vi "TCP Client_33.vi"(0 "CMD":i32(ring) items=["OCP_IF_CMD_TRACE_READ", "OCP_IF_CMD_TRACE_RESET", "OCP_IF_CMD_TRACE_GET_SIZE", "OCP_IF_CMD_TRACE_SET_SIZE", "OCP_IF_CMD_TRACE_GET_NUMBER_SIGNALS", "OCP_IF_CMD_TRACE_GET_SIGNALS_NAMES", "OCP_IF_CMD_TRACE_GET_NUMBER_TRACES", "OCP_IF_CMD_TRACE_GET_TRACES_NAMES", "OCP_IF_CMD_TRACE_GET_ADDRESS", "OCP_IF_CMD_CS_STATUS", "OCP_IF_CMD_CS_ENABLE", "OCP_IF_CMD_CS_DISABLE", "OCP_IF_CMD_CS_CONTROLLER_IF", "OCP_IF_CMD_CS_HARDWARE_IF", "OCP_IF_CMD_CS_GET_NUMBER_CONTROLLERS", "OCP_IF_CMD_CS_GET_CONTROLLERS_NAMES", "OCP_IF_CMD_PLATFORM_ID", "OCP_IF_CMD_PLATFORM_IF", "OCP_IF_CMD_OPIL_UPDATE_MEASUREMENTS", "OCP_IF_CMD_OPIL_UPDATE_SIM_DATA", "OCP_IF_CMD_OPIL_RUN_CONTROL", "OCP_IF_CMD_OPIL_INITIALIZE_CONTROL", "OCP_IF_CMD_OPIL_GET_CONTROL", "OCP_IF_CMD_OPIL_GET_CONTROLLER_DATA", "OCP_IF_CMD_END"], 2 "Input Cluster":T3, 3 "error in (no error)":errorcluster, 8 "Comunication Cluster":T1) -> (6 "Output cluster":T2, 7 "R_message 1":string, 10 "error out":errorcluster)   [LabVIEW 2021]
uses:
  <vilib>/ErrorRing/Error Ring.xnode
  <vilib>/Utility/error.llb/Error Cluster From Error Code.vi
panel:
  out "R_Data string length":cluster{i32}
  out "W_Data string length: \nbytes written 2":i32
  out "W_Data string_flat":string
  # "0-> OCP_IF_CMD_TRACE_READ = 0, //LV: SIZE - CMD - ID || RESPONSE: SIZE - DATA\n1->\tOCP_IF_CMD_TRACE_RESET, //SIZE - CMD - ID || RESPONSE: SIZE\n2-> OCP_IF_CMD_TRACE_GET_SIZE, //SIZE - CMD - ID || RESPONSE: SIZE - TRACE_SIZE (4 bztes)\n3->\tOCP_IF_CMD_TRACE_SET_SIZE, //SIZE - CMD - ID - TRACE_SIZE ( 4 bytes) || RESPONSE: SIZE\n4->\tOCP_IF_CMD_TRACE_GET_NUMBER_SIGNALS, //SIZE - CMD - ID || RESPONSE: SIZE - NB_SIGNALS (4 bytes)\n5->\tOCP_IF_CMD_TRACE_GET_SIGNALS_NAMES, //SIZE - CMD - ID || RESPONSE: SIZE - string\n6->\tOCP_IF_CMD_TRACE_GET_NUMBER_TRACES, //SIZE - CMD  || RESPONSE: SIZE - NB_TRACES (4 bytes)\n7->\tOCP_IF_CMD_TRACE_GET_TRACES_NAMES, //SIZE - CMD || RESPONSE: SIZE - NB_TRACES (N bytes)\n8-> OCP_IF_CMD_TRACE_GET_ADDRESS, //SIZE - CMD - ID || RESPONSE: SIZE - TRACE ADDRESS (4 bytes)\n9-> OCP_IF_CMD_CS_STATUS, //SIZE - CMD - ID || RESPONSE: SIZE - CS STATUS (4 bytes)\n10-> OCP_IF_CMD_CS_ENABLE, //SIZE - CMD - ID || RESPONSE: SIZE\n11-> OCP_IF_CMD_CS_DISABLE, //SIZE - CMD - ID || RESPONSE: SIZE\n12-> OCP_IF_CMD_CS_CONTROLLER_IF, //SIZE - CMD - ID - DATA (N) || RESPONSE: SIZE - DATA (M)\n13-> OCP_IF_CMD_CS_HARDWARE_IF, //SIZE - CMD - ID - DATA (N) || RESPONSE: SIZE - DATA (M)\n14-> OCP_IF_CMD_CS_GET_NUMBER_CONTROLLERS, //SIZE - CMD || RESPONSE: SIZE - NB CSs\n15-> OCP_IF_CMD_CS_GET_CONTROLLERS_NAMES, //SIZE - CMD || RESPONSE: SIZE - string NAMES CSs"
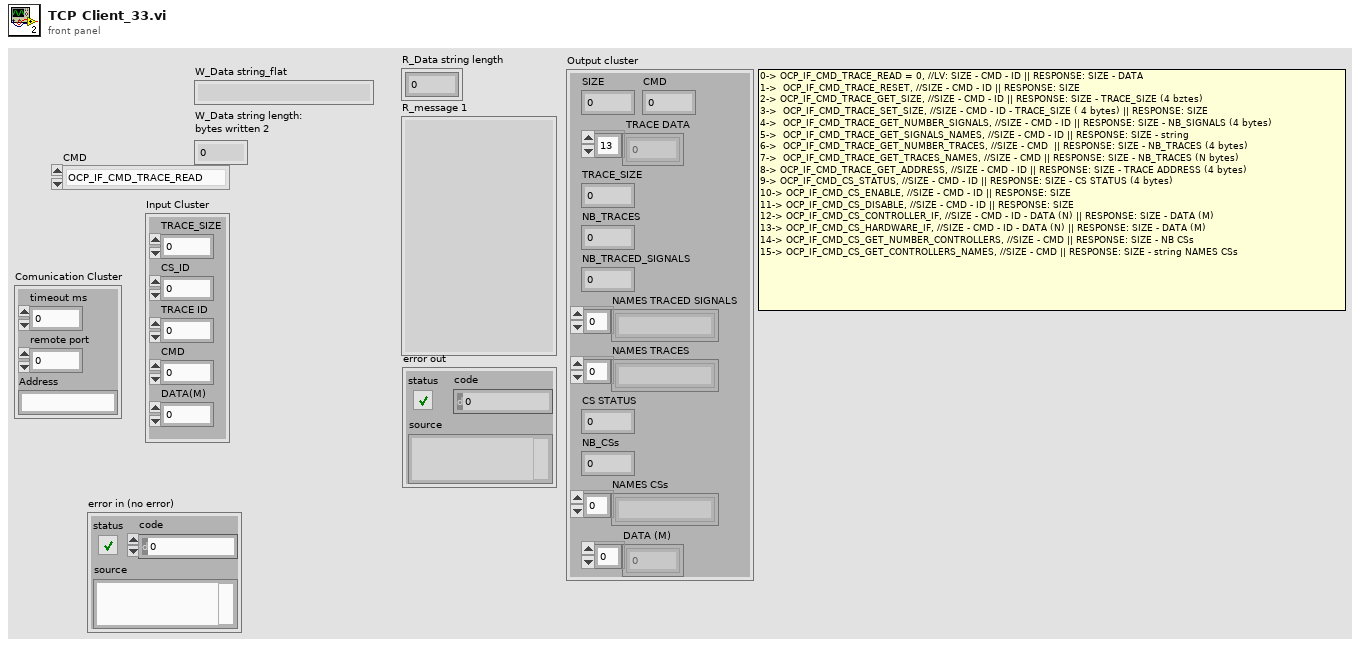
[diagram p1: front panel]
types:
  T1 = cluster{"timeout ms":i32, "remote port":u16, "Address":string}
  T2 = cluster{"SIZE":i32, " TRACE DATA":sgl[], "TRACE_SIZE":i32, "NB_TRACES":i32, "NB_TRACED_SIGNALS":i32, "NAMES TRACED SIGNALS":string[], "NAMES TRACES":string[], "CS STATUS":i32, "NB_CSs":i32, "NAMES CSs":string[], "DATA (M)":sgl[], "CMD":i32}
  T3 = cluster{"TRACE_SIZE":i32, "CS_ID":i32, "TRACE ID":i32, "CMD":i32, "DATA(M)":i32}
  T4 = enum16{"big-endian, network order", "native, host order", "little-endian"}
  T5 = enum16{"Standard", "Buffered", "CRLF", "Immediate"}
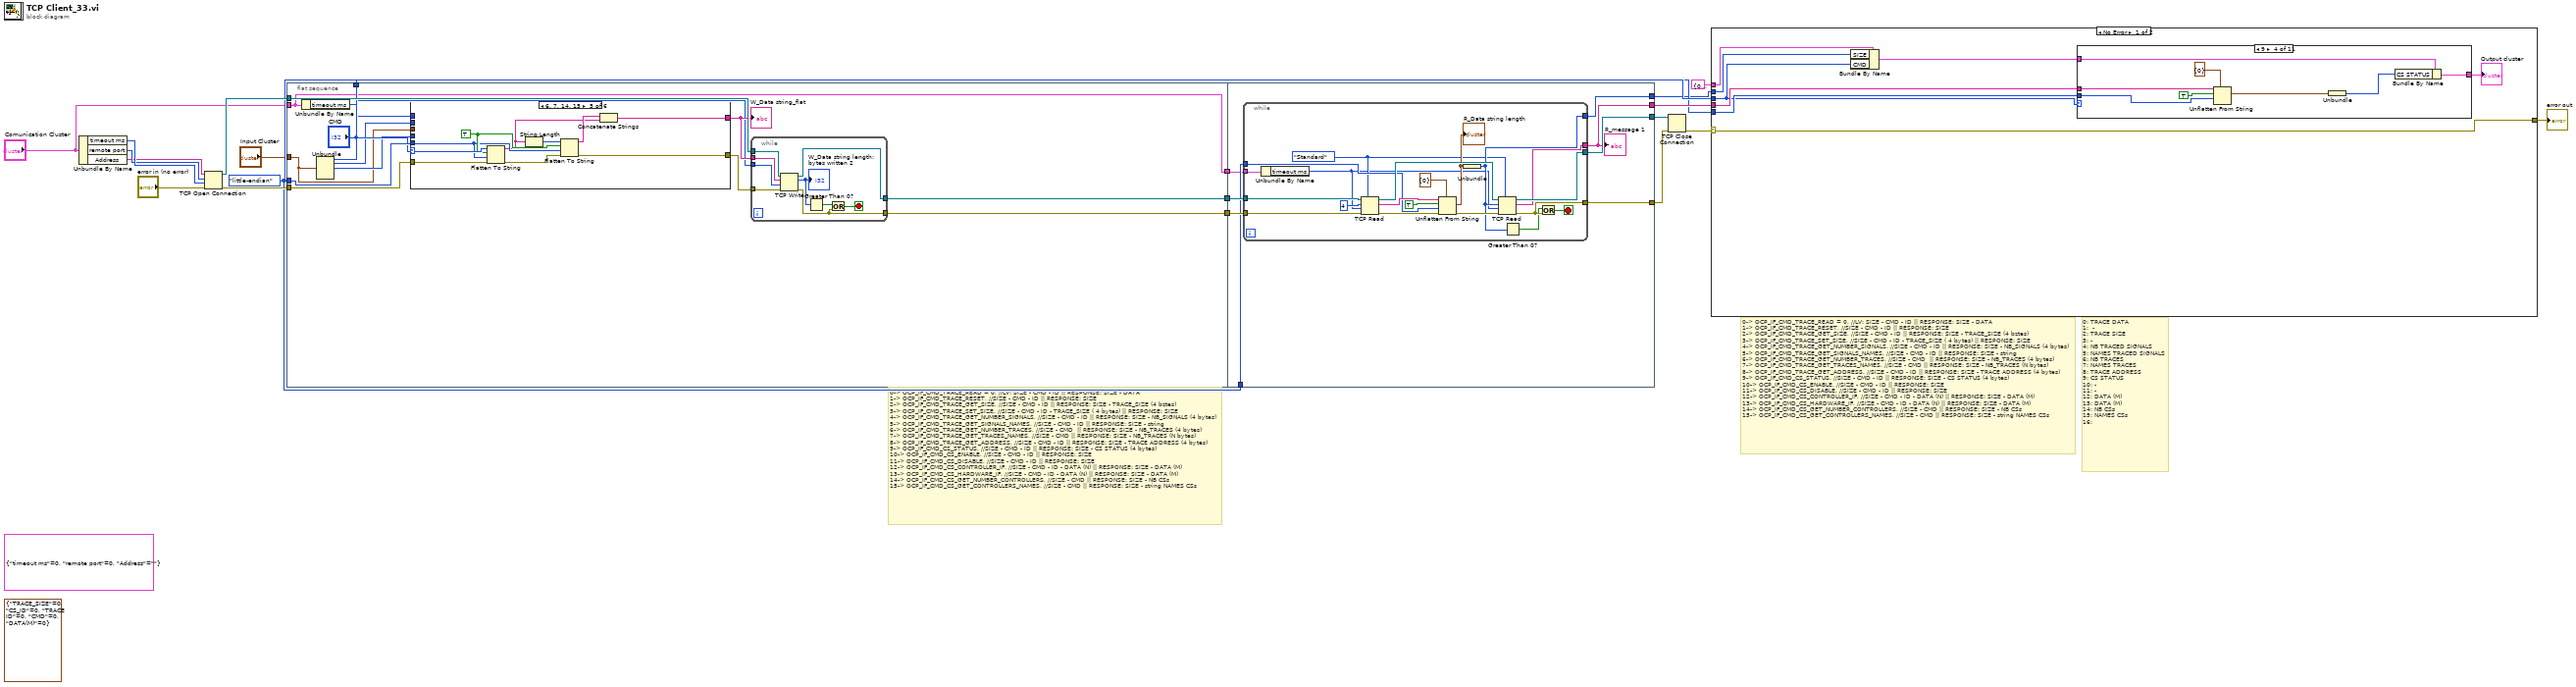
[diagram p0: block diagram]
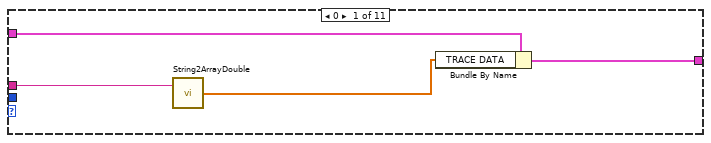
[diagram p2: hidden frame]
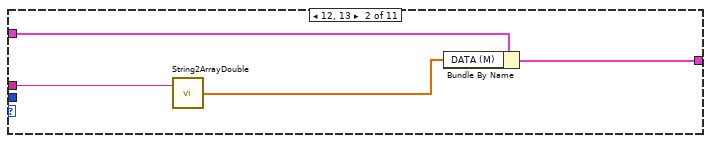
[diagram p3: hidden frame]
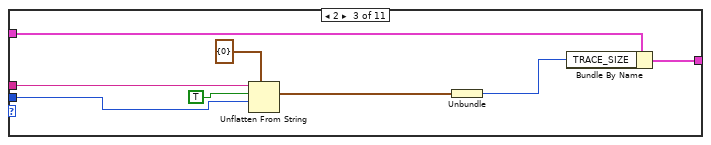
[diagram p4: hidden frame]
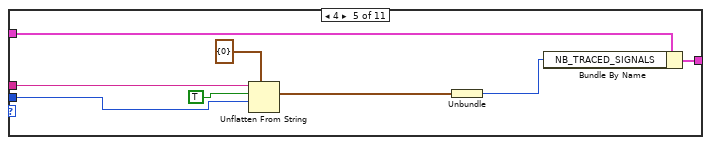
[diagram p5: hidden frame]
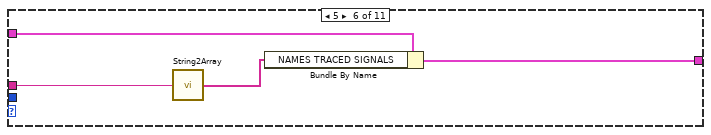
[diagram p6: hidden frame]
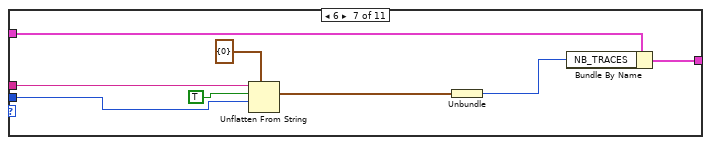
[diagram p7: hidden frame]
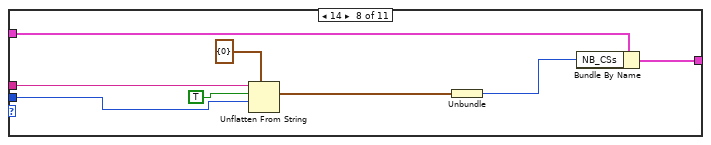
[diagram p8: hidden frame]
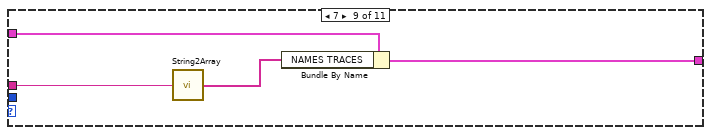
[diagram p9: hidden frame]
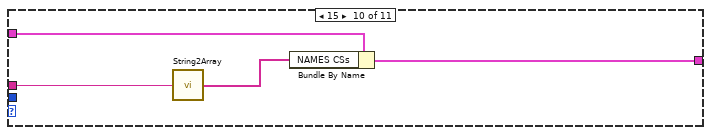
[diagram p10: hidden frame]
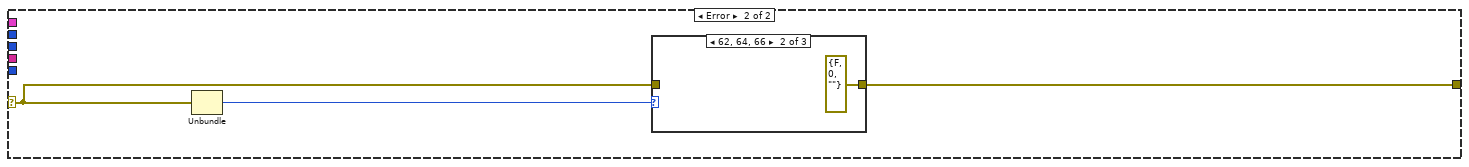
[diagram p12: hidden frame]
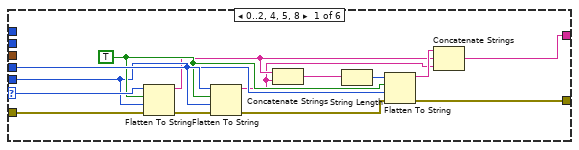
[diagram p15: hidden frame]
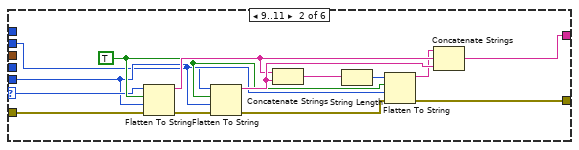
[diagram p16: hidden frame]
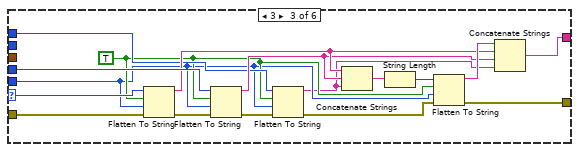
[diagram p17: hidden frame]
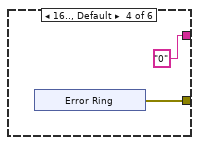
[diagram p18: hidden frame]
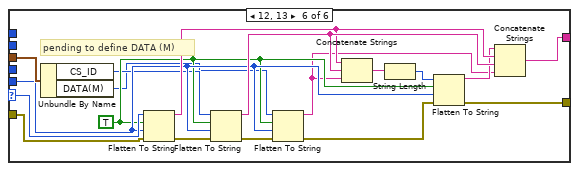
[diagram p19: hidden frame]
diagram:
  (unwired) T1 {"timeout ms"=0, "remote port"=0, "Address"=""}
  (unwired) T3 {"TRACE_SIZE"=0, "CS_ID"=0, "TRACE ID"=0, "CMD"=0, "DATA(M)"=0}
  w8 = T4."little-endian" ("byte order (0:big-endian, network order)")
  # "0-> OCP_IF_CMD_TRACE_READ = 0, //LV: SIZE - CMD - ID || RESPONSE: SIZE - DATA\n1->\tOCP_IF_CMD_TRACE_RESET, //SIZE - CMD - ID || RESPONSE: SIZE\n2-> OCP_IF_CMD_TRACE_GET_SIZE, //SIZE - CMD - ID || RESPONSE: SIZE - TRACE_SIZE (4 bztes)\n3->\tOCP_IF_CMD_TRACE_SET_SIZE, //SIZE - CMD - ID - TRACE_SIZE ( 4 bytes) || RESPONSE: SIZE\n4->\tOCP_IF_CMD_TRACE_GET_NUMBER_SIGNALS, //SIZE - CMD - ID || RESPONSE: SIZE - NB_SIGNALS (4 bytes)\n5->\tOCP_IF_CMD_TRACE_GET_SIGNALS_NAMES, //SIZE - CMD - ID || RESPONSE: SIZE - string\n6->\tOCP_IF_CMD_TRACE_GET_NUMBER_TRACES, //SIZE - CMD  || RESPONSE: SIZE - NB_TRACES (4 bytes)\n7->\tOCP_IF_CMD_TRACE_GET_TRACES_NAMES, //SIZE - CMD || RESPONSE: SIZE - NB_TRACES (N bytes)\n8-> OCP_IF_CMD_TRACE_GET_ADDRESS, //SIZE - CMD - ID || RESPONSE: SIZE - TRACE ADDRESS (4 bytes)\n9-> OCP_IF_CMD_CS_STATUS, //SIZE - CMD - ID || RESPONSE: SIZE - CS STATUS (4 bytes)\n10-> OCP_IF_CMD_CS_ENABLE, //SIZE - CMD - ID || RESPONSE: SIZE\n11-> OCP_IF_CMD_CS_DISABLE, //SIZE - CMD - ID || RESPONSE: SIZE\n12-> OCP_IF_CMD_CS_CONTROLLER_IF, //SIZE - CMD - ID - DATA (N) || RESPONSE: SIZE - DATA (M)\n13-> OCP_IF_CMD_CS_HARDWARE_IF, //SIZE - CMD - ID - DATA (N) || RESPONSE: SIZE - DATA (M)\n14-> OCP_IF_CMD_CS_GET_NUMBER_CONTROLLERS, //SIZE - CMD || RESPONSE: SIZE - NB CSs\n15-> OCP_IF_CMD_CS_GET_CONTROLLERS_NAMES, //SIZE - CMD || RESPONSE: SIZE - string NAMES CSs"
  # "0: TRACE DATA\n1:  -\n2: TRACE SIZE\n3: -\n4: NB TRACED SIGNALS\n5: NAMES TRACED SIGNALS\n6: NB TRACES\n7: NAMES TRACES\n8: TRACE ADDRESS\n9: CS STATUS\n10: -\n11: -\n12: DATA (M)\n13: DATA (M)\n14: NB CSs \n15: NAMES CSs \n16:"
  # "0-> OCP_IF_CMD_TRACE_READ = 0, //LV: SIZE - CMD - ID || RESPONSE: SIZE - DATA\n1->\tOCP_IF_CMD_TRACE_RESET, //SIZE - CMD - ID || RESPONSE: SIZE\n2-> OCP_IF_CMD_TRACE_GET_SIZE, //SIZE - CMD - ID || RESPONSE: SIZE - TRACE_SIZE (4 bztes)\n3->\tOCP_IF_CMD_TRACE_SET_SIZE, //SIZE - CMD - ID - TRACE_SIZE ( 4 bytes) || RESPONSE: SIZE\n4->\tOCP_IF_CMD_TRACE_GET_NUMBER_SIGNALS, //SIZE - CMD - ID || RESPONSE: SIZE - NB_SIGNALS (4 bytes)\n5->\tOCP_IF_CMD_TRACE_GET_SIGNALS_NAMES, //SIZE - CMD - ID || RESPONSE: SIZE - string\n6->\tOCP_IF_CMD_TRACE_GET_NUMBER_TRACES, //SIZE - CMD  || RESPONSE: SIZE - NB_TRACES (4 bytes)\n7->\tOCP_IF_CMD_TRACE_GET_TRACES_NAMES, //SIZE - CMD || RESPONSE: SIZE - NB_TRACES (N bytes)\n8-> OCP_IF_CMD_TRACE_GET_ADDRESS, //SIZE - CMD - ID || RESPONSE: SIZE - TRACE ADDRESS (4 bytes)\n9-> OCP_IF_CMD_CS_STATUS, //SIZE - CMD - ID || RESPONSE: SIZE - CS STATUS (4 bytes)\n10-> OCP_IF_CMD_CS_ENABLE, //SIZE - CMD - ID || RESPONSE: SIZE\n11-> OCP_IF_CMD_CS_DISABLE, //SIZE - CMD - ID || RESPONSE: SIZE\n12-> OCP_IF_CMD_CS_CONTROLLER_IF, //SIZE - CMD - ID - DATA (N) || RESPONSE: SIZE - DATA (M)\n13-> OCP_IF_CMD_CS_HARDWARE_IF, //SIZE - CMD - ID - DATA (N) || RESPONSE: SIZE - DATA (M)\n14-> OCP_IF_CMD_CS_GET_NUMBER_CONTROLLERS, //SIZE - CMD || RESPONSE: SIZE - NB CSs\n15-> OCP_IF_CMD_CS_GET_CONTROLLERS_NAMES, //SIZE - CMD || RESPONSE: SIZE - string NAMES CSs"
  n1 = Unbundle By Name("Comunication Cluster") -> ("timeout ms"=w4:i32, "remote port"=w3:u16, "Address"=w2:string)
  n2 = TCP Open Connection(address=w2, remote port or service name=w3, timeout ms (60000)=w4, error in (no error)="error in (no error)") -> (connection ID=w20:refnum<k5>, error out=w19:errorcluster)  [unwired: 1 in]
  n3 = flat-sequence {
    tunnel: w20 -> [w34]
    tunnel: w19 -> [w31]
    tunnel: [w33] -> w18
    tunnel: [w32] -> w17
    tunnel: w8 -> [w30]
    tunnel: ["CMD"] -> w11
    tunnel: "Input Cluster" -> [w24]
    tunnel: "Comunication Cluster" -> [w22]
    tunnel: [w22] -> w1
    tunnel: w18 -> [w131]
    tunnel: w17 -> [w130]
    tunnel: [w129] -> w14
    tunnel: [w128] -> w13
    tunnel: w8 -> [w127]
    tunnel: [w126] -> w10
    tunnel: [w125] -> w7
    tunnel: w1 -> [w124]
    frame #0 {
      n4 = Unbundle By Name(w22) -> ("timeout ms"=w23:i32)
      n5 = Unbundle(w24) -> ("TRACE_SIZE"=w25:i32, "CS_ID"=w27:i32, "TRACE ID"=w26:i32)  [unwired: 2 out]
      n6 = case shown="6, 7, 14, 15" "CMD" {
        selector: "CMD" -> [w55 w62 w86 _ w104 w115]
        tunnel: w31 -> [w57 w63 w88 _ w105 w114]
        tunnel: w30 -> [w48 w61 w74 _ w100 w111]
        tunnel: w26 -> [w54 _ w85 _ _ _]
        tunnel: [w47 w59 w81 "0" w99 w117] -> w29
        tunnel: [w46 w58 w73 w90 w97 w116] -> w21
        tunnel: w25 -> [_ _ w76 _ _ _]
        tunnel: w27 -> [_ w60 _ _ _ _]
        tunnel: w24 -> [_ _ _ _ _ w113]
        frame 0..2, 4, 5, 8 {
          w49 = TRUE ("prepend array or string size? (T)")
          n7 = Flatten To String(anything=w55, prepend array or string size? (T)=w49, byte order (0:big-endian, network order)=w48, error in (no error)=w57) -> (data string=w45:string, error out=w56:errorcluster)  [unwired: 1 out]
          n8 = Flatten To String(anything=w54, prepend array or string size? (T)=w49, byte order (0:big-endian, network order)=w48, error in (no error)=w56) -> (data string=w44:string, error out=w51:errorcluster)  [unwired: 1 out]
          n9 = Concatenate Strings(w45, w44) -> (w53:string)
          n10 = String Length(string=w53) -> (length=w52:i32)
          n11 = Flatten To String(anything=w52, prepend array or string size? (T)=w49, byte order (0:big-endian, network order)=w48, error in (no error)=w51) -> (data string=w50:string, error out=w46:errorcluster)  [unwired: 1 out]
          n12 = Concatenate Strings(w50, w45, w44) -> (w47:string)
        }
        frame 9..11 {
          w64 = TRUE ("prepend array or string size? (T)")
          n13 = Flatten To String(anything=w62, prepend array or string size? (T)=w64, byte order (0:big-endian, network order)=w61, error in (no error)=w63) -> (data string=w70:string, error out=w65:errorcluster)  [unwired: 1 out]
          n14 = Flatten To String(anything=w60, prepend array or string size? (T)=w64, byte order (0:big-endian, network order)=w61, error in (no error)=w65) -> (data string=w71:string, error out=w68:errorcluster)  [unwired: 1 out]
          n15 = Concatenate Strings(w70, w71) -> (w66:string)
          n16 = String Length(string=w66) -> (length=w67:i32)
          n17 = Flatten To String(anything=w67, prepend array or string size? (T)=w64, byte order (0:big-endian, network order)=w61, error in (no error)=w68) -> (data string=w69:string, error out=w58:errorcluster)  [unwired: 1 out]
          n18 = Concatenate Strings(w69, w70, w71) -> (w59:string)
        }
        frame 3 {
          w75 = TRUE ("prepend array or string size? (T)")
          n19 = Flatten To String(anything=w86, prepend array or string size? (T)=w75, byte order (0:big-endian, network order)=w74, error in (no error)=w88) -> (data string=w80:string, error out=w87:errorcluster)  [unwired: 1 out]
          n20 = Flatten To String(anything=w85, prepend array or string size? (T)=w75, byte order (0:big-endian, network order)=w74, error in (no error)=w87) -> (data string=w79:string, error out=w78:errorcluster)  [unwired: 1 out]
          n21 = Flatten To String(anything=w76, prepend array or string size? (T)=w75, byte order (0:big-endian, network order)=w74, error in (no error)=w78) -> (data string=w72:string, error out=w77:errorcluster)  [unwired: 1 out]
          n22 = Concatenate Strings(w80, w79, w72) -> (w84:string)
          n23 = String Length(string=w84) -> (length=w83:i32)
          n24 = Flatten To String(anything=w83, prepend array or string size? (T)=w75, byte order (0:big-endian, network order)=w74, error in (no error)=w77) -> (data string=w82:string, error out=w73:errorcluster)  [unwired: 1 out]
          n25 = Concatenate Strings(w82, w80, w79, w72) -> (w81:string)
        }
        frame 16.., Default {
          n26 = xnode "Error Ring"() -> ("error out"=w90:errorcluster)
        }
        frame 6, 7, 14, 15 {
          w101 = TRUE ("prepend array or string size? (T)")
          n27 = Flatten To String(anything=w104, prepend array or string size? (T)=w101, byte order (0:big-endian, network order)=w100, error in (no error)=w105) -> (data string=w96:string, error out=w98:errorcluster)  [unwired: 1 out]
          n28 = String Length(string=w96) -> (length=w103:i32)
          n29 = Flatten To String(anything=w103, prepend array or string size? (T)=w101, byte order (0:big-endian, network order)=w100, error in (no error)=w98) -> (data string=w102:string, error out=w97:errorcluster)  [unwired: 1 out]
          n30 = Concatenate Strings(w102, w96) -> (w99:string)
        }
        frame 12, 13 {
          w110 = TRUE ("prepend array or string size? (T)")
          # "pending to define DATA (M)"
          n31 = Unbundle By Name(w113) -> ("CS_ID"=w109:i32, "DATA(M)"=w108:i32)
          n32 = Flatten To String(anything=w115, prepend array or string size? (T)=w110, byte order (0:big-endian, network order)=w111, error in (no error)=w114) -> (data string=w122:string, error out=w118:errorcluster)  [unwired: 1 out]
          n33 = Flatten To String(anything=w109, prepend array or string size? (T)=w110, byte order (0:big-endian, network order)=w111, error in (no error)=w118) -> (data string=w123:string, error out=w112:errorcluster)  [unwired: 1 out]
          n34 = Flatten To String(anything=w108, prepend array or string size? (T)=w110, byte order (0:big-endian, network order)=w111, error in (no error)=w112) -> (data string=w107:string, error out=w106:errorcluster)  [unwired: 1 out]
          n35 = Concatenate Strings(w122, w123, w107) -> (w119:string)
          n36 = String Length(string=w119) -> (length=w120:i32)
          n37 = Flatten To String(anything=w120, prepend array or string size? (T)=w110, byte order (0:big-endian, network order)=w111, error in (no error)=w106) -> (data string=w121:string, error out=w116:errorcluster)  [unwired: 1 out]
          n38 = Concatenate Strings(w121, w122, w123, w107) -> (w117:string)
        }
      }
      "W_Data string_flat" <- w29
      n39 = while {
        tunnel: w29 -> [w41]
        tunnel: w23 -> [w40]
        tunnel: w21 -> [w39]
        tunnel: [w37] -> w33
        tunnel: w34 -> [w43]
        tunnel: [w42] -> w32
        stop <- w38 stop-if-true
        n40 = TCP Write(connection ID=w43, data in=w41, error in (no error)=w39, 9:w40) -> (connection ID out=w42:refnum<k5>, bytes written=w36:i32, error out=w37:errorcluster)
        "W_Data string length: \nbytes written 2" <- w36
        n41 = Greater Than 0?(x=w36) -> (x > 0?=w35:bool)
        n42 = Or(x=w35, y=w37) -> (x .or. y?=w38:bool)
      }
    }
    frame #1 {
      n43 = while {
        tunnel: w127 -> [w141]
        tunnel: [w139] -> w126
        tunnel: [w136] -> w125
        tunnel: w130 -> [w149]
        tunnel: [w148] -> w129
        tunnel: w131 -> [w150]
        tunnel: [w138] -> w128
        tunnel: w124 -> [w132]
        stop <- w137 stop-if-true
        w134 = T5."Standard" ("mode (standard)")
        n44 = Unbundle By Name(w132) -> ("timeout ms"=w133:i32)
        n45 = TCP Read(connection ID=w149, bytes to read=4, error in (no error)=w150, 7:w134, 9:w133) -> (connection ID out=w151:refnum<k5>, data out=w147:string, error out=w143:errorcluster)
        n46 = Unflatten From String(type=cluster{i32} {0}, binary string=w147, data includes array or string size? (T)=TRUE, byte order (0:big-endian, network order)=w141, error in (no error)=w143) -> (value=w144:cluster{i32}, error out=w142:errorcluster)  [unwired: 1 out]
        "R_Data string length" <- w144
        n47 = Unbundle(w144) -> (w136:i32)
        n48 = TCP Read(connection ID=w151, bytes to read=w136, error in (no error)=w142, 7:w134, 9:w133) -> (connection ID out=w148:refnum<k5>, data out=w139:string, error out=w138:errorcluster)
        n49 = Greater Than 0?(x=w136) -> (x > 0?=w135:bool)
        n50 = Or(x=w135, y=w138) -> (x .or. y?=w137:bool)
      }
      "R_message 1" <- w126
    }
  }
  n51 = TCP Close Connection(connection ID=w14, error in (no error)=w13) -> (error out=w15:errorcluster)  [unwired: 1 in, 1 out]
  n52 = case shown="No Error" w15 {
    selector: w15 -> [w159 w222]
    tunnel: [w159 w221] -> w16
    tunnel: w11 -> [w153 _]
    tunnel: w10 -> [w155 _]
    tunnel: T2 {"SIZE"=0, " TRACE DATA"=[], "TRACE_SIZE"=0, "NB_TRACES"=0, "NB_TRACED_SIGNALS"=0, "NAMES TRACED SIGNALS"=[], "NAMES TRACES"=[], "CS STATUS"=0, "NB_CSs"=0, "NAMES CSs"=[], "DATA (M)"=[], "CMD"=0} ("input cluster") -> [w158 _]
    tunnel: w8 -> [w154 _]
    tunnel: w7 -> [w156 _]
    frame No Error {
      n53 = Bundle By Name(cluster=w158, "SIZE"=w156, "CMD"=w153) -> (w157:T2)
      n54 = case shown="9" w153 {
        tunnel: [w162 w166 w174 w182 w190 w194 w203 w211 w214 w218 w220] -> w152
        tunnel: w157 -> [w163 w167 w175 w183 w191 w195 w200 w208 w215 w219 w220]
        tunnel: w155 -> [w160 w164 w172 w180 w187 w193 w198 w206 w213 w217 _]
        tunnel: w154 -> [_ _ w170 w178 w186 _ w199 w207 _ _ _]
        frame 0 {
          n55 = call "String2ArrayDouble.vi"("R_message 1"=w160) -> ("Array"=w161:sgl[])  [unwired: 1 in]
          n56 = Bundle By Name(cluster=w163, "TRACE DATA"=w161) -> (w162:T2)
        }
        frame 12, 13 {
          n57 = call "String2ArrayDouble.vi"("R_message 1"=w164) -> ("Array"=w165:sgl[])  [unwired: 1 in]
          n58 = Bundle By Name(cluster=w167, "DATA (M)"=w165) -> (w166:T2)
        }
        frame 2 {
          n59 = Unflatten From String(type=cluster{i32} {0}, binary string=w172, data includes array or string size? (T)=TRUE, byte order (0:big-endian, network order)=w170) -> (value=w169:cluster{i32})  [unwired: 1 in, 2 out]
          n60 = Unbundle(w169) -> (w168:i32)
          n61 = Bundle By Name(cluster=w175, "TRACE_SIZE"=w168) -> (w174:T2)
        }
        frame 9 {
          n62 = Unflatten From String(type=cluster{i32} {0}, binary string=w180, data includes array or string size? (T)=TRUE, byte order (0:big-endian, network order)=w178) -> (value=w177:cluster{i32})  [unwired: 1 in, 2 out]
          n63 = Unbundle(w177) -> (w176:i32)
          n64 = Bundle By Name(cluster=w183, "CS STATUS"=w176) -> (w182:T2)
        }
        frame 4 {
          n65 = Unflatten From String(type=cluster{i32} {0}, binary string=w187, data includes array or string size? (T)=TRUE, byte order (0:big-endian, network order)=w186) -> (value=w188:cluster{i32})  [unwired: 1 in, 2 out]
          n66 = Unbundle(w188) -> (w184:i32)
          n67 = Bundle By Name(cluster=w191, "NB_TRACED_SIGNALS"=w184) -> (w190:T2)
        }
        frame 5 {
          n68 = call "String2Array.vi"("R_message 1"=w193) -> ("Array 2"=w192:string[])
          n69 = Bundle By Name(cluster=w195, "NAMES TRACED SIGNALS"=w192) -> (w194:T2)
        }
        frame 6 {
          n70 = Unflatten From String(type=cluster{i32} {0}, binary string=w198, data includes array or string size? (T)=TRUE, byte order (0:big-endian, network order)=w199) -> (value=w202:cluster{i32})  [unwired: 1 in, 2 out]
          n71 = Unbundle(w202) -> (w196:i32)
          n72 = Bundle By Name(cluster=w200, "NB_TRACES"=w196) -> (w203:T2)
        }
        frame 14 {
          n73 = Unflatten From String(type=cluster{i32} {0}, binary string=w206, data includes array or string size? (T)=TRUE, byte order (0:big-endian, network order)=w207) -> (value=w210:cluster{i32})  [unwired: 1 in, 2 out]
          n74 = Unbundle(w210) -> (w204:i32)
          n75 = Bundle By Name(cluster=w208, "NB_CSs"=w204) -> (w211:T2)
        }
        frame 7 {
          n76 = call "String2Array.vi"("R_message 1"=w213) -> ("Array 2"=w212:string[])
          n77 = Bundle By Name(cluster=w215, "NAMES TRACES"=w212) -> (w214:T2)
        }
        frame 15 {
          n78 = call "String2Array.vi"("R_message 1"=w217) -> ("Array 2"=w216:string[])
          n79 = Bundle By Name(cluster=w219, "NAMES CSs"=w216) -> (w218:T2)
        }
        frame 8, Default {
        }
      }
      "Output cluster" <- w152
    }
    frame Error {
      n80 = Unbundle(w222) -> ("code"=w223:i32)  [unwired: 2 out]
      n81 = case shown="62, 64, 66" w223 {
        tunnel: [w224 errorcluster {"status"=FALSE, "code"=0, "source"=""} ("error IO") w226] -> w221
        tunnel: w222 -> [w224 _ w226]
        frame 0, Default {
        }
        frame 62, 64, 66 {
        }
        frame 56 {
        }
      }
    }
  }
  "error out" <- w16
